vi "gmmregTransformLowLevel.vi"(0 "nctrlpts":i32, 1 "coordCtrlPts":dbl[](array[numeric]), 2 "npts":i32, 3 "coord":dbl[](array[numeric]), 4 "nout":i32, 5 "out":dbl[](array[numeric]), 6 "param0":dbl[](array[numeric]), 7 "normParams":dbl[](array[numeric]), 8 "dim":i32, 9 "denormParams":dbl[](array[numeric])) -> (11 "denormParams out":dbl[](array[numeric]), 12 "param0 out":dbl[](array[numeric]), 13 "normParams out":dbl[](array[numeric]), 15 "coordCtrlPts out":dbl[](array[numeric]), 17 "coord out":dbl[](array[numeric]), 19 "out out":dbl[](array[numeric]))   [LabVIEW 2017]
uses:
  dll/wormUtilities/x64/Release/wormUtilities.dll
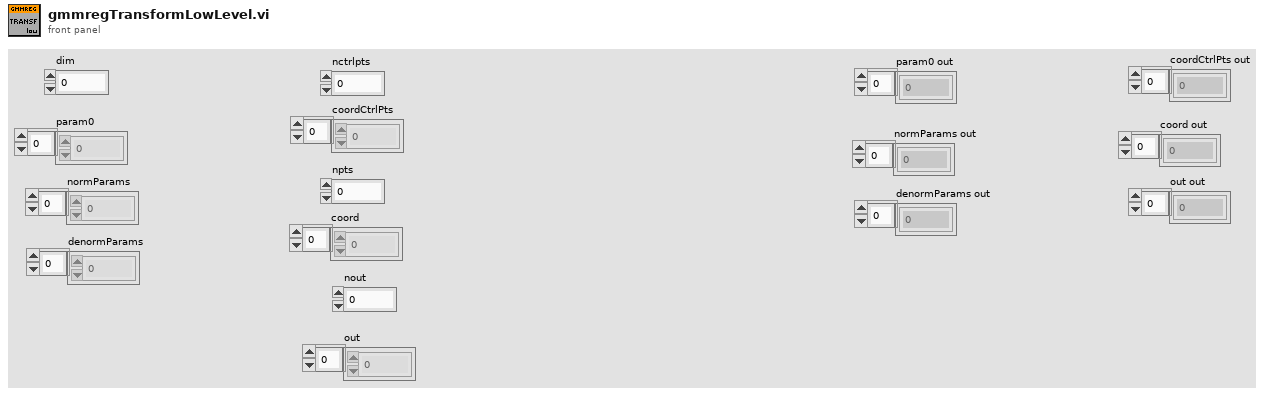
[diagram p1: front panel]
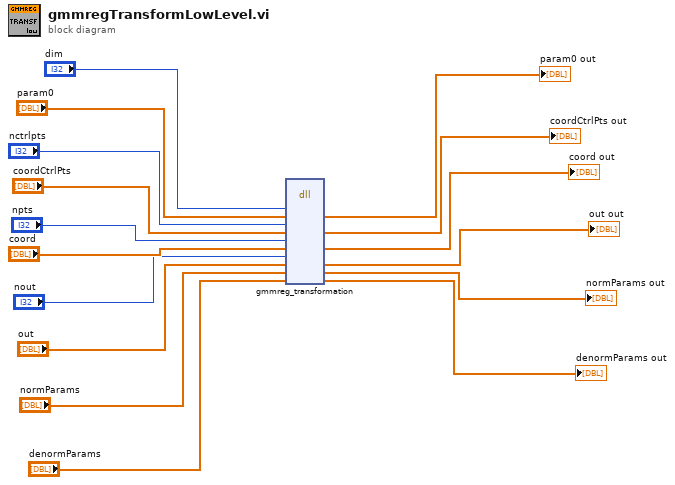
[diagram p0: block diagram]
diagram:
  n1 = dll-call lib="C:/Users/francesco/dev/pump-probe/dll/wormUtilities/x64/Release/wormUtilities.dll" fn="gmmreg_transformation"("dim"="dim", "param0"="param0", "nctrlpts"="nctrlpts", "coordCtrlPts"="coordCtrlPts", "npts"="npts", "coord"="coord", "nout"="nout", "out"="out", "normParams"="normParams", "denormParams"="denormParams") -> ("param0"=→"param0 out":dbl[], "coordCtrlPts"=→"coordCtrlPts out":dbl[], "coord"=→"coord out":dbl[], "out"=→"out out":dbl[], "normParams"=→"normParams out":dbl[], "denormParams"=→"denormParams out":dbl[])  [unwired: 8 in, 2 out]
